vi "Palindromic Word Detector.vi"() -> ()   [LabVIEW 2017]
panel:
  out "Palindrome?":bool
  in  "Word":string
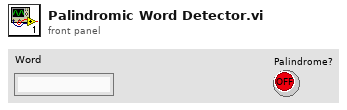
[diagram p1: front panel]
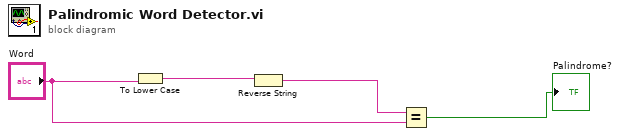
[diagram p0: block diagram]
diagram:
  n1 = To Lower Case(string="Word") -> (all lower case string=w2:string)
  n2 = Reverse String(1:w2) -> (0:w4:string)
  n3 = Equal?(x=w4, y="Word") -> (x = y?=→"Palindrome?":bool)
